vi "Record Period.vi"(8 "error in (no error)":errorcluster, 10 "Record Period":u16(ring)=9 items=["1 Millisecond", "2 Milliseconds", "5 Milliseconds", "10 Milliseconds", "20 Milliseconds", "50 Milliseconds", "100 Milliseconds", "200 Milliseconds", "500 Milliseconds", "1 Second", "2 Seconds", "5 Seconds", "10 Seconds", "20 Seconds", "1 Minute", "2 Minutes", "5 Minutes", "10 Minutes", "20 Minutes"], 11 "VISA resource name":refnum<visa-resource-name>) -> (0 "error out":errorcluster, 3 "VISA resource name out":refnum<visa-resource-name>)   [LabVIEW 2017, in "Sefram DAS220.lvlib"]
doc: "Set the record period on the device."
uses:
  <instrlib>/Sefram DAS220/Sefram DAS220.lvlib
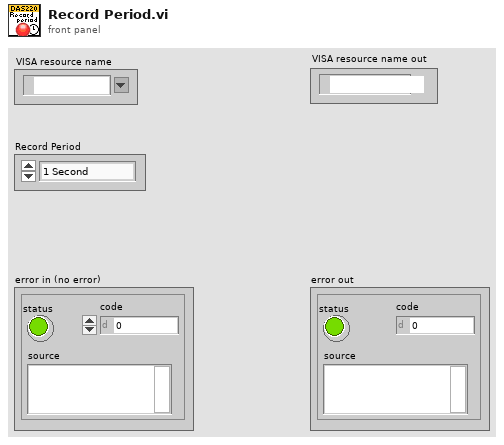
[diagram p1: front panel]
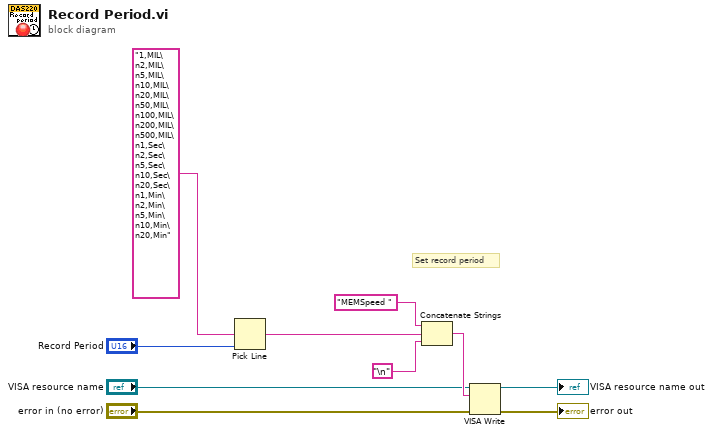
[diagram p0: block diagram]
diagram:
  # "Set record period"
  n1 = Pick Line(multi-line string="1,MIL\n2,MIL\n5,MIL\n10,MIL\n20,MIL\n50,MIL\n100,MIL\n200,MIL\n500,MIL\n1,Sec\n2,Sec\n5,Sec\n10,Sec\n20,Sec\n1,Min\n2,Min\n5,Min\n10,Min\n20,Min", line index="Record Period") -> (output string=w4:string)  [unwired: 1 in]
  n2 = Concatenate Strings("MEMSpeed " ("string"), w4, "\n") -> (w10:string)
  n3 = VISA Write(VISA resource name="VISA resource name", write buffer=w10, error in (no error)="error in (no error)") -> (VISA resource name out=→"VISA resource name out":refnum<visa-resource-name>, error out=→"error out":errorcluster)  [unwired: 1 out]
